vi "Generate Dictionary.vi"(6 "Fonts":T1[](array[typedef]), 7 "Additional Languages":string[](array[string]), 8 "error in (no error)":errorcluster, 9 "Current VI Language":string, 10 "Dictionary Path":path, 11 "VIs in":refnum<vi>[](array[refnum])) -> (0 "error out":errorcluster)   [LabVIEW 2017, in "JKI Simple Localization.lvlib"]
uses:
  JKI Simple Localization.lvlib
  Definitions/Private/FontCluster.ctl
  Definitions/Dictionary--Cluster.ctl
  Definitions/Private/Phrase Dictionary.ctl
  <vilib>/addons/_JKI.lib/Serialization/JSON/JKI JSON Serialization.lvlib
panel:
  out "Text Written (for debug)":string
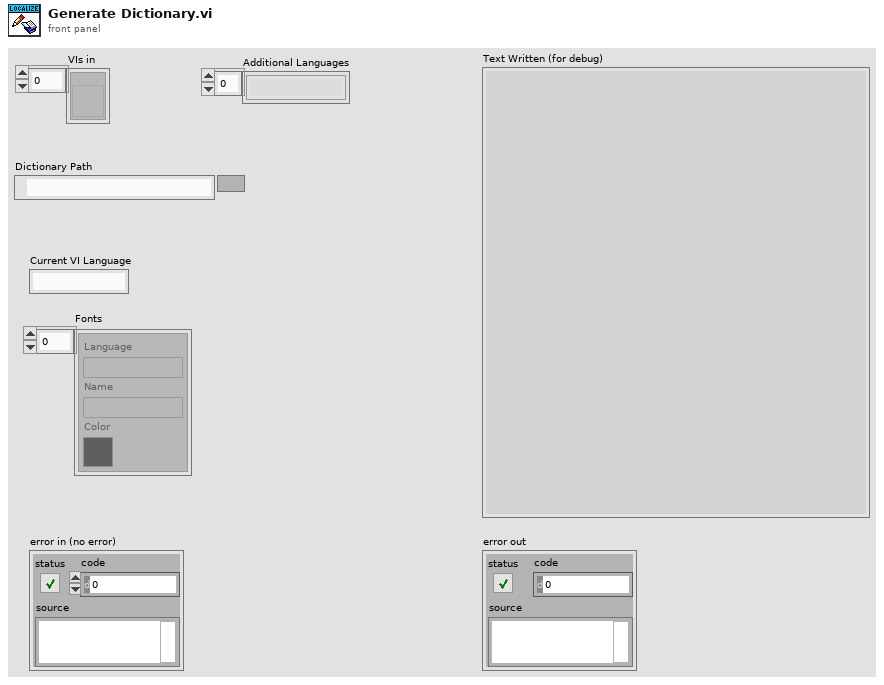
[diagram p1: front panel]
types:
  T1 = typedef "JKI Simple Localization.lvlib/FontCluster.ctl" = cluster{"Language":string, "Name":string, "Color":u32}
  T2 = typedef "JKI Simple Localization.lvlib/Dictionary--Cluster.ctl" = cluster{"Languages":string[], "Fonts":T1[], "Phrase Dictionary":T3[]}
  T3 = typedef "JKI Simple Localization.lvlib/Phrase Dictionary.ctl" = cluster{"Key":string, "Phrases":string[]}
  T4 = enum16{"open", "replace", "create", "open or create", "replace or create", "replace or create with confirmation"}
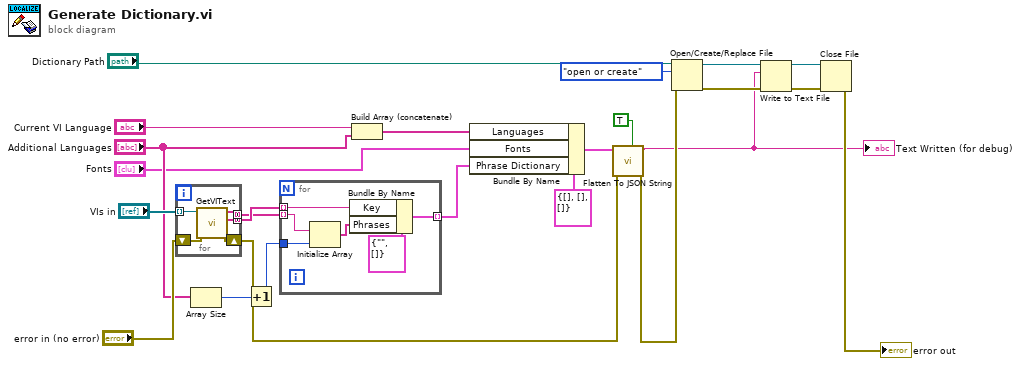
[diagram p0: block diagram]
diagram:
  n1 = for {
    tunnel: "VIs in" -> [w28] mode=indexing
    tunnel: [w27] -> w15 mode=concatenating
    tunnel: [w26] -> w14 mode=concatenating
    shift-right: [w25] -> w3
    shift-left: "error in (no error)" -> [w29]
    n2 = call "GetVIText.vi"("error in (no error)"=w29, "VI"=w28) -> ("error out"=w25:errorcluster, "Control UIDs"=w27:string[], "Control Text"=w26:string[])  [unwired: 7 in]
  }
  n3 = Array Size(array="Additional Languages") -> (size(s)=w13:i32)
  n4 = Increment(x=w13) -> (x+1=w12:i32)
  n5 = for {
    tunnel: w15 -> [w34] mode=indexing
    tunnel: w14 -> [w32] mode=indexing
    tunnel: w12 -> [w33]
    tunnel: [w30] -> w6 mode=indexing
    n6 = Initialize Array(w32, w33) -> (w31:string[])
    n7 = Bundle By Name(cluster=T3 {"Key"="", "Phrases"=[]} ("Phrase Dictionary"), "Key"=w34, "Phrases"=w31) -> (w30:T3)
  }
  n8 = Build Array (concatenate)("Current VI Language", "Additional Languages") -> (w8:string[])
  n9 = Bundle By Name(cluster=T2 {"Languages"=[], "Fonts"=[], "Phrase Dictionary"=[]} ("Localization"), "Languages"=w8, "Fonts"="Fonts", "Phrase Dictionary"=w6) -> (w4:T2)
  n10 = call <vilib>:"Flatten To JSON String.vi"("Numeric Extensions (F)"=TRUE, "error in (no error)"=w3, "Variant"=w4) -> ("error out"=w2:errorcluster, "JSON String"=w1:string)  [unwired: 7 in]
  "Text Written (for debug)" <- w1
  n11 = Open/Create/Replace File(file path (use dialog)="Dictionary Path", error in=w2, operation (0:open)=T4."open or create") -> (refnum out=w19:refnum<file>, error out=w21:errorcluster)  [unwired: 3 in, 1 out]
  n12 = Write to Text File(file (use dialog)=w19, text=w1, error in=w21) -> (refnum out=w23:refnum<file>, error out=w22:errorcluster)  [unwired: 1 in, 1 out]
  n13 = Close File(refnum=w23, error in=w22) -> (error out=→"error out":errorcluster)  [unwired: 1 out]
